vi "Shooter.vi"(1 "Run":bool, 2 "Enum":enum16{"Start", "Run", "End"}(ring)) -> ()   [LabVIEW 2014]
uses:
  TypeDefs/PWM Module 1.ctl
  <vilib>/Rock Robotics/SystemInterfaces/Typedef/FPGA_TypedefDigitalModule.ctl
  <vilib>/Rock Robotics/SystemInterfaces/DIO/FPGA_DIOPWMChannel.ctl
  <vilib>/Rock Robotics/SystemInterfaces/DIO/FPGA_DIORelayChannel.ctl
  <vilib>/Rock Robotics/WPI/SafetyOutput/WPI_SafetyOutputConfigMenu.ctl
  <vilib>/Rock Robotics/WPI/MotorControl/WPI_MotorControlOpen Victor.vi
panel:
  in  "Power":dbl=-1.0 format="%#_13g"
  in  "PWM Module (DIO A)":T1={"Module"=enum."Digital Module 1", "Roller"=enum."PWM 1", "Right Drive 3"=enum."PWM 2", "Right Drive 2"=enum."PWM 3", "Right Drive 1"=enum."PWM 4", "Shooter"=enum."PWM 5", "Unassigned"=enum."PWM 6", "Unassigned"=enum."PWM 7", "Left Drive 1"=enum."PWM 8", "Left Drive 2"=enum."PWM 9", "Left Drive 3"=enum."PWM 9", "Unassigned"=enum."Relay 1", "Unassigned"=enum."Relay 2", "Unassigned"=enum."Relay 3", "Unassigned"=enum."Relay 3", "Unassigned"=enum."Invalid", "Unassigned"=enum."Relay 1", "Unassigned"=enum."Relay 1", "Compressor "=enum."Relay 1"}
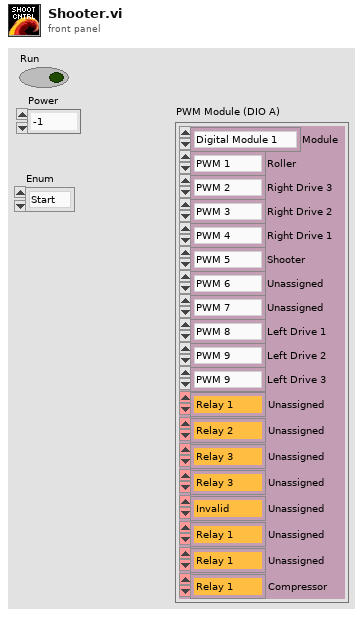
[diagram p1: front panel]
types:
  T1 = typedef "PWM Module 1.ctl" = cluster{"Module":T2, "Roller":T3, "Right Drive 3":T3, "Right Drive 2":T3, "Right Drive 1":T3, "Shooter":T3, "Unassigned":T3, "Unassigned":T3, "Left Drive 1":T3, "Left Drive 2":T3, "Left Drive 3":T3, "Unassigned":T4, "Unassigned":T4, "Unassigned":T4, "Unassigned":T4, "Unassigned":T4, "Unassigned":T4, "Unassigned":T4, "Compressor ":T4}
  T2 = typedef "FPGA_TypedefDigitalModule.ctl" = enum16{"Digital Module 1", "Digital Module 2"}
  T3 = typedef "FPGA_DIOPWMChannel.ctl" = enum8{"PWM 1", "PWM 2", "PWM 3", "PWM 4", "PWM 5", "PWM 6", "PWM 7", "PWM 8", "PWM 9", "PWM 10", "Invalid"}
  T4 = typedef "FPGA_DIORelayChannel.ctl" = enum8{"Relay 1", "Relay 2", "Relay 3", "Relay 4", "Relay 5", "Relay 6", "Relay 7", "Relay 8", "Invalid"}
  T5 = typedef "WPI_SafetyOutputConfigMenu.ctl" = enum16{"Enable", "Disable"}
  T6 = typedef "WPI_MotorControlDeviceRef.ctl" = cluster{"DeviceStatus":errorcluster, "Type":enum16{"PWM", "CAN"}, "PWM":cluster{"Digital Module":T2, "PWM Channel":T3, "DeadBand":T7}, "CAN":cluster{"Device Number":u8, "Control Mode":T8, "Semaphore":T9, "Max Vout":dbl}, "Invert":bool, "TransformRef":T10, "InvTransformRef":T10}
  T7 = typedef "WPI_PWMDeadband.ctl" = cluster{"Name":string, "maxPositivePwm":i32, "minPositivePwm":i32, "centerPwm":i32, "maxNegativePwm":i32, "minNegativePwm":i32, "angularRange":u16}
  T8 = typedef "WPI_CANJaguar_ControlMode.ctl" = enum8{"Percent VBus", "Current", "Speed", "Position", "Voltage"}
  T9 = typedef "Semaphore RefNum" = refnum<k1>
  T10 = typedef "WPI_PWMTransform_ConPane.ctl" = refnum<vi>
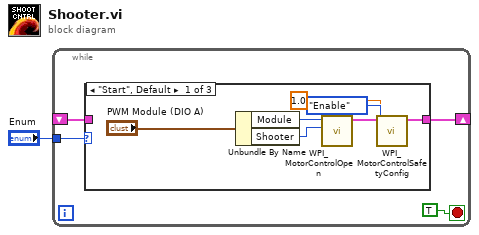
[diagram p0: block diagram]
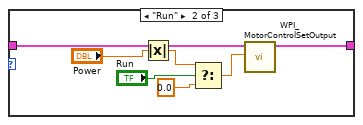
[diagram p2: hidden frame]
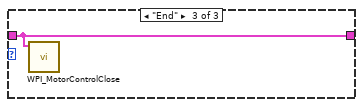
[diagram p3: hidden frame]
diagram:
  n1 = while {
    tunnel: "Enum" -> [w4]
    shift-right: [w2] -> _
    shift-left: _ -> [w3]
    stop <- TRUE stop-if-true
    n2 = case shown="\"Start\", Default" w4 {
      tunnel: w3 -> [_ w19 w20]
      tunnel: [w8 w18 w20] -> w2
      frame "Start", Default {
        n3 = Unbundle By Name("PWM Module (DIO A)") -> ("Module"=w11:T2, "Shooter"=w10:T3)
        n4 = call-poly <vilib>:"WPI_MotorControlOpen.vi"("PWM Channel"=w10, "Digital Module (Module 1)"=w11) -> ("MotorControlDeviceRef"=w9:T6)  [unwired: 8 in, 1 out]
        n5 = call <vilib>:"WPI_MotorControlSafetyConfig.vi"("timeout (s)"=1.0, "mode"=WPI_SafetyOutputConfigMenu."Enable", "MotorControlDevRef"=w9) -> ("MotorControlDevRef"=w8:T6)  [unwired: 7 in, 1 out]
      }
      frame "Run" {
        n6 = Absolute Value(x="Power") -> (abs(x)=w13:dbl)
        n7 = Select(t=w13, s="Run", f=0.0) -> (s? t:f=w17:dbl)
        n8 = call <vilib>:"WPI_MotorControlSetOutput.vi"("Output"=w17, "MotorControlDevRef"=w19) -> ("MotorControlDevRef"=w18:T6)  [unwired: 7 in, 2 out]
      }
      frame "End" {
        n9 = call <vilib>:"WPI_MotorControlClose.vi"("MotorControlDevRef"=w20) -> ()  [unwired: 10 in, 1 out]
      }
    }
  }
